vi "Numeric String to Digits.vi"(0 "Numeric String":string, 1 "Ignore:F Include:T Spelled Numbers? (F)":bool, 2 "Ignore:F Include:T Overlapped Spelled Numbers? (F)":bool) -> (3 "Digits":i32[](array[numeric]))   [LabVIEW 2020]
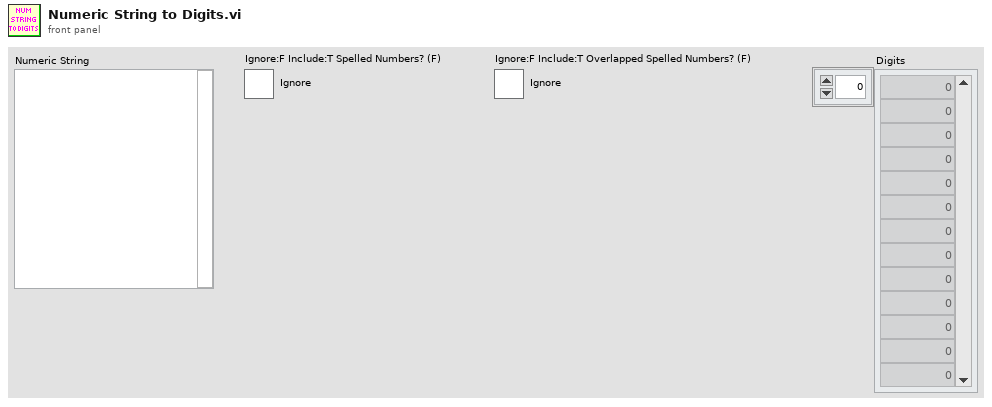
[diagram p1: front panel]
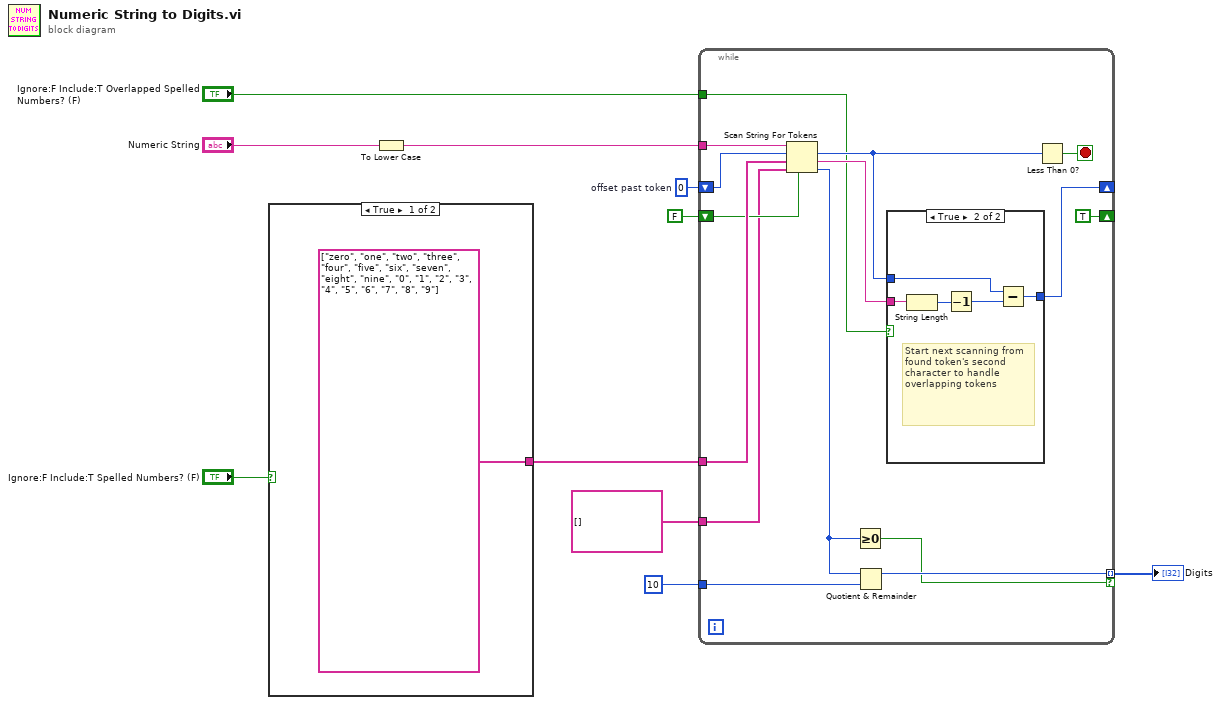
[diagram p0: block diagram]
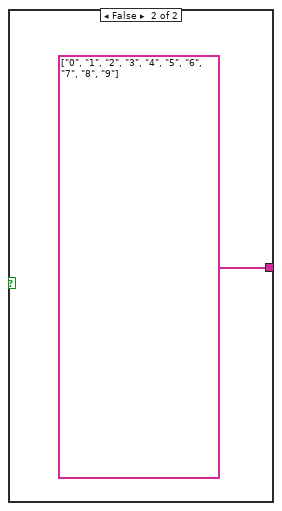
[diagram p2: hidden frame]
diagram:
  w7 = 0  # offset past token
  n1 = case shown="True" "Ignore:F Include:T Spelled Numbers? (F)" {
    tunnel: [string[] ["zero", "one", "two", "three", "four", "five", "six", "seven", "eight", "nine", "0", "1", "2", "3", "4", "5", "6", "7", "8", "9"] string[] ["0", "1", "2", "3", "4", "5", "6", "7", "8", "9"]] -> w8
    frame True {
    }
    frame False {
    }
  }
  n2 = To Lower Case(string="Numeric String") -> (all lower case string=w9:string)
  n3 = while {
    tunnel: w8 -> [w25]
    shift-right: [w15] -> _
    shift-left: w7 -> [w26]
    tunnel: [w23] -> w6 mode=indexing if=w18
    tunnel: w9 -> [w27]
    shift-right: [TRUE] -> _
    shift-left: FALSE -> [w22]
    tunnel: string[] [] -> [w20]
    tunnel: 10 -> [w19]
    tunnel: "Ignore:F Include:T Overlapped Spelled Numbers? (F)" -> [w13]
    stop <- w24 stop-if-true
    n4 = Scan String For Tokens(4:w22, 6:w20, 7:w25, 8:w26, 9:w27) -> (0:w17:i32, 1:w16:string, 2:w14:i32)  [unwired: 1 in, 1 out]
    n5 = Greater Or Equal To 0?(x=w17) -> (x >= 0?=w18:bool)
    n6 = Quotient & Remainder(x=w17, y=w19) -> (x-y*floor(x/y)=w23:i32)  [unwired: 1 out]
    n7 = case shown="True" w13 {
      tunnel: w16 -> [_ w33]
      tunnel: [w28 w30] -> w15
      tunnel: w14 -> [w28 w29]
      frame False {
      }
      frame True {
        # "Start next scanning from found token's second character to handle overlapping tokens"
        n8 = String Length(string=w33) -> (length=w32:i32)
        n9 = Decrement(x=w32) -> (x-1=w31:i32)
        n10 = Subtract(x=w29, y=w31) -> (x-y=w30:i32)
      }
    }
    n11 = Less Than 0?(x=w14) -> (x < 0?=w24:bool)
  }
  "Digits" <- w6
